vi "Punkt aus Tabelle lesen.vi"(9 "Index":i32, 11 "Stufen Tabelle":T1) -> (0 "Sollwert":sgl, 1 "Sollwert":string, 2 "Punkt":i32, 3 "Punkt":string)   [LabVIEW 2020, in "Linearisierung v2.lvlib"]
uses:
  Linearisierung v2.lvlib
  Gasteiler/Stufen Tabelle.ctl
  Gasteiler/Gasteiler.lvlib
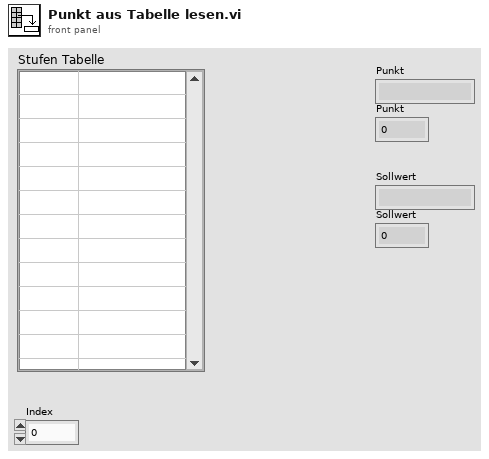
[diagram p1: front panel]
types:
  T1 = typedef "Linearisierung v2.lvlib/Gasteiler.lvlib/Stufen Tabelle.ctl" = string[][]
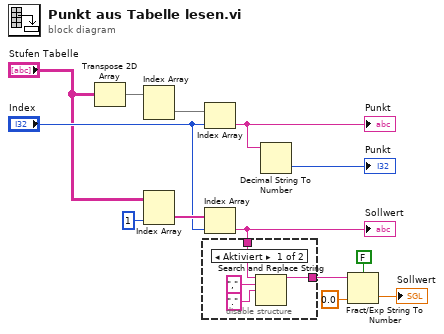
[diagram p0: block diagram]
diagram:
  n1 = Transpose 2D Array(2D array="Stufen Tabelle") -> (transposed array=w7:T1)
  n2 = Index Array(array=w7) -> (element=w13:string[])  [unwired: 2 in]
  n3 = Index Array(array="Stufen Tabelle", index (col)=1 ("Deaktivierter Index (Spalte)")) -> (element=w11:string[])  [unwired: 1 in]
  n4 = Index Array(array=w13, index="Index") -> (element=w6:string)
  "Punkt" <- w6
  n5 = Index Array(array=w11, index="Index") -> (element=w1:string)
  "Sollwert" <- w1
  n6 = disable-structure shown="Aktiviert" {
    disable-tunnel: [w15 w18] -> w2
    disable-tunnel: w1 -> [w14 w18]
    frame Enabled {
      n7 = Search and Replace String(input string=w14, search string="," ("Such-String"), replace string="." ("String ersetzen(\"\")")) -> (result string=w15:string)  [unwired: 5 in, 3 out]
    }
    frame Disabled {
    }
  }
  n8 = Decimal String To Number(string=w6) -> (number=→"Punkt":i32)  [unwired: 2 in, 1 out]
  n9 = Fract/Exp String To Number(use system decimal point (T)=FALSE ("Systemdezimalzeichen verwenden (T)"), string=w2, default (0 dbl)=sgl 0.0 ("Standard (0 I32)")) -> (number=→"Sollwert":sgl)  [unwired: 1 in, 1 out]
